vi "visual object recognition.vi"() -> ()   [LabVIEW 2019]
uses:
  <vilib>/vision/driver/NI_Vision_Acquisition_Software.lvlib
  <vilib>/vision/driver/IMAQdx.llb/IMAQdx Acquisition Mode.ctl
  Control 1.ctl
  <vilib>/vision/driver/IMAQdx.llb/IMAQdx Buffer Number Mode.ctl
  <vilib>/userDefined/High Color/IMAQdx.ctl
  <vilib>/vision/Image Controls.llb/IMAQ Image.ctl
panel:
  out "?":T1
  in  "analysis":bool
  out "image path":path
  out "snap shot":T2
  in  "Snap":bool
  out "Image":T2 caption="Image Out"
  out "Frame rate":dbl
  out "Buffer Number":u32
  in  "stop":bool
  in  "module path":path
  in  "Python version":string
  in  "Camera":T3
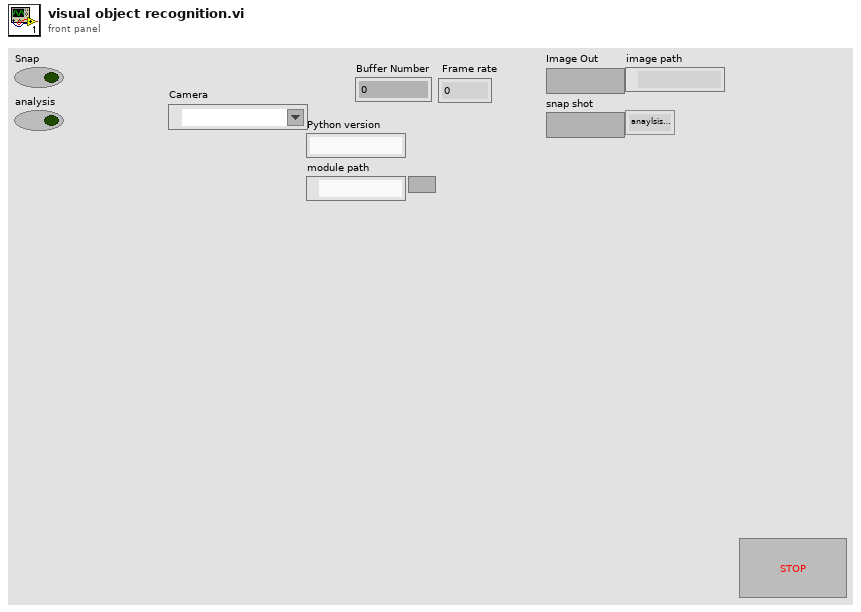
[diagram p1: front panel]
types:
  T1 = typedef "Control 1.ctl" = enum16{"anaylsis using python", "acquire image"}
  T2 = typedef "IMAQ Image.ctl" = refnum<image>
  T3 = typedef "IMAQdx.ctl" = refnum<k21>
  T4 = typedef "NI_Vision_Acquisition_Software.lvlib/IMAQdx Acquisition Mode.ctl" = enum32{"One Shot", "Continuous"}
  T5 = typedef "NI_Vision_Acquisition_Software.lvlib/IMAQdx Buffer Number Mode.ctl" = enum32{"Next", "Last", "Buffer Number", "Every", "Last New"}
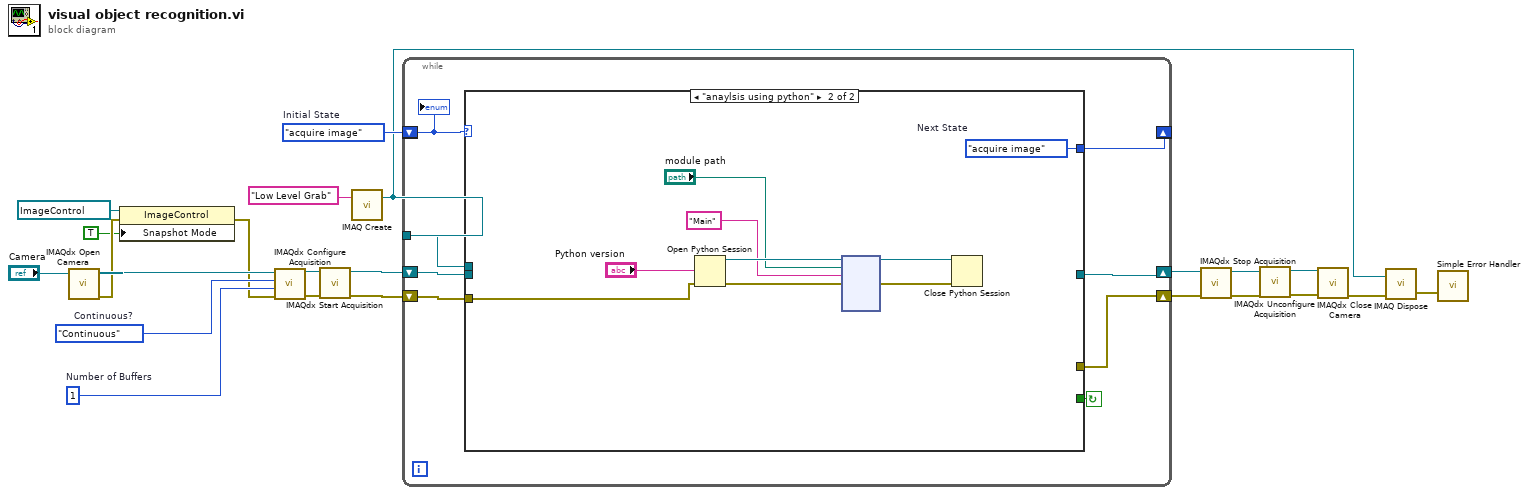
[diagram p0: block diagram]
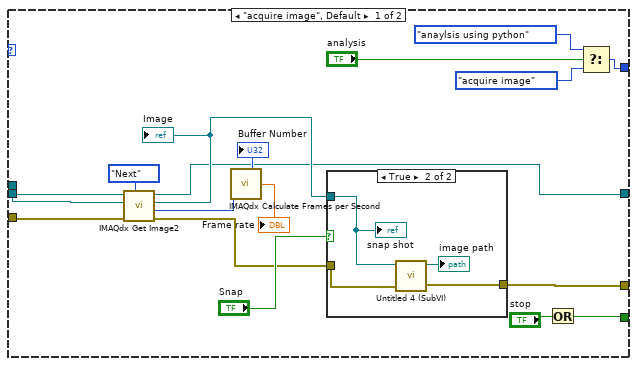
[diagram p2: hidden frame]
diagram:
  w6 = Control_1."acquire image"  # Initial State
  w15 = u32 1  # Number of Buffers
  w16 = IMAQdx_Acquisition_Mode."Continuous"  # Continuous?
  n1 = call <vilib>:"IMAQdx Open Camera.vi"("Session In"="Camera") -> ("error out"=w5:errorcluster, "Session Out"=w19:T3)  [unwired: 2 in, 7 out]
  n2 = property class="ImageControl"(reference=refnum<vi> refnum, error in=w5, "Snapshot Mode"=TRUE) -> (error out=w4:errorcluster)  [unwired: 1 out]
  n3 = call <vilib>:"IMAQdx Configure Acquisition.vi"("error in"=w4, "Number of Buffers"=w15, "Continuous?"=w16, "Session In"=w19) -> ("error out"=w17:errorcluster, "Session Out"=w18:T3)  [unwired: 6 in]
  n4 = call <vilib>:"IMAQdx Start Acquisition.vi"("error in"=w17, "Session In"=w18) -> ("error out"=w20:errorcluster, "Session Out"=w21:T3)  [unwired: 8 in]
  n5 = call "IMAQ Create"("Image Name"="Low Level Grab") -> ("New Image"=w1:T2)  [unwired: 3 in, 2 out]
  n6 = while {
    tunnel: w1 -> [w30]
    shift-right: [w27] -> w10
    shift-left: _ -> [_]
    shift-right: [w26] -> w9
    shift-left: _ -> [_]
    shift-right: _ -> [_]
    shift-left: w20 -> [w28]
    shift-right: _ -> [_]
    shift-left: w21 -> [w29]
    shift-right: [w24] -> _
    shift-left: _ -> [_]
    shift-right: _ -> [_]
    shift-left: w6 -> [w25]
    stop <- w31 continue-if-true
    n7 = case shown="\"anaylsis using python\"" w25 {
      tunnel: [w44 _] -> w31
      tunnel: w30 -> [w46 _]
      tunnel: w29 -> [w45 _]
      tunnel: w28 -> [w47 w55]
      tunnel: [w32 _] -> w27
      tunnel: [w37 _] -> w26
      tunnel: [w35 w54] -> w24
      frame "acquire image", Default {
        n8 = call <vilib>:"IMAQdx Get Image2.vi"("Buffer Number Mode (Next)"=IMAQdx_Buffer_Number_Mode."Next", "error in"=w47, "Image In"=w46, "Session In"=w45) -> ("error out"=w38:errorcluster, "Buffer Number Out"=w43:u32, "Image Out"=w40:T2, "Session Out"=w32:T3)  [unwired: 4 in]
        "Image" <- w40
        n9 = call <vilib>:"IMAQdx Calculate Frames per Second.vi"("Frames per Second Update Interval (ms)"=w43) -> ("Processed Frames per Second"=→"Frame rate":dbl, "Images Missed"=→"Buffer Number":u32)  [unwired: 8 in, 5 out]
        n10 = case shown="True" "Snap" {
          tunnel: w40 -> [_ w52]
          tunnel: w38 -> [_ w53]
          tunnel: [_ w51] -> w37
          frame False {
          }
          frame True {
            n11 = call "Untitled 4 (SubVI).vi"("error in (no error)"=w53, "Refnum in"=w52) -> ("error out"=w51:errorcluster, "image path"=→"image path":path)  [unwired: 8 in]
            "snap shot" <- w52
          }
        }
        n12 = Or(y="stop") -> (x .or. y?=w44:bool)  [unwired: 1 out]
        n13 = Select(t=Control_1."anaylsis using python", s="analysis", f=Control_1."acquire image") -> (s? t:f=w35:T1)
      }
      frame "anaylsis using python" {
        w54 = Control_1."acquire image"  # Next State
        n14 = Open Python Session(python version="Python version", 3:w55) -> (session out=w62:refnum<k35>, error out=w61:errorcluster)  [unwired: 1 in]
        n15 = node(w62, "module path", "Main" ("function name"), w61) -> (w59:refnum<k35>, w58:errorcluster)  [unwired: 6 in, 2 out]
        n16 = Close Python Session(session in=w59, error in=w58) -> ()  [unwired: 1 out]
      }
    }
    "?" <- w25
  }
  n17 = call <vilib>:"IMAQdx Stop Acquisition.vi"("error in"=w9, "Session In"=w10) -> ("error out"=w14:errorcluster, "Session Out"=w12:T3)  [unwired: 8 in]
  n18 = call <vilib>:"IMAQdx Unconfigure Acquisition.vi"("error in"=w14, "Session In"=w12) -> ("error out"=w13:errorcluster, "Session Out"=w11:T3)  [unwired: 8 in]
  n19 = call <vilib>:"IMAQdx Close Camera.vi"("error in"=w13, "Session In"=w11) -> ("error out"=w8:errorcluster)  [unwired: 9 out]
  n20 = call "IMAQ Dispose"("Image"=w1, "error in (no error)"=w8) -> ("error out"=w7:errorcluster)  [unwired: 4 in]
  n21 = call <vilib>:"Simple Error Handler.vi"("error in (no error)"=w7) -> ()  [unwired: 1 in, 8 out]
